vi "Delay with Cancel.vi"(8 "error in (no error)":errorcluster, 9 "Delay (ms)":u32) -> (0 "error out":errorcluster, 1 "Elaplsed":u32)   [LabVIEW 2018]
uses:
  Main/Main Globals.vi
  Utilities.lvlib
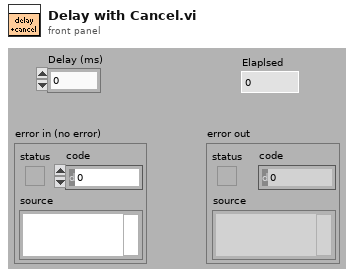
[diagram p1: front panel]
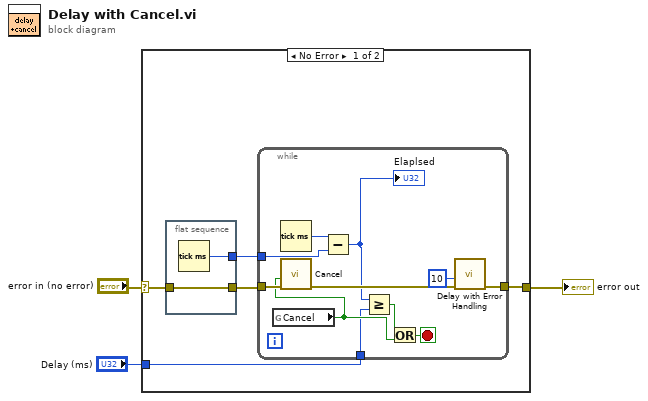
[diagram p0: block diagram]
diagram:
  n1 = case shown="No Error" "error in (no error)" {
    selector: "error in (no error)" -> [w8 w22]
    tunnel: [w4 w22] -> w2
    tunnel: "Delay (ms)" -> [w5 _]
    frame No Error {
      n2 = flat-sequence {
        tunnel: w8 -> [w10]
        tunnel: [w10] -> w7
        tunnel: [w9] -> w6
        frame #0 {
          n3 = Tick Count (ms)() -> (millisecond timer value=w9:u32)
        }
      }
      n4 = while {
        tunnel: w7 -> [w20]
        tunnel: [w15] -> w4
        tunnel: w6 -> [w17]
        tunnel: w5 -> [w13]
        stop <- w21 stop-if-true
        n5 = global read "Main Globals.vi" "Cancel"() -> (w19:bool)
        n6 = Tick Count (ms)() -> (millisecond timer value=w18:u32)
        n7 = call "Cancel.vi"("error in (no error)"=w20, "Cancel"=w19) -> ("error out"=w16:errorcluster)  [unwired: 9 in]
        n8 = Subtract(x=w18, y=w17) -> (x-y=w14:u32)
        "Elaplsed" <- w14
        n9 = Greater Or Equal?(x=w14, y=w13) -> (x >= y?=w12:bool)
        n10 = Or(x=w12, y=w19) -> (x .or. y?=w21:bool)
        n11 = call "Delay with Error Handling.vi"("error in (no error)"=w16, "Delay (ms)"=u32 10) -> ("error out"=w15:errorcluster)  [unwired: 9 in]
      }
    }
    frame Error {
    }
  }
  "error out" <- w2
